vi "Write Numeric.vi"(8 "error in (no error)":errorcluster, 10 "Numeric":dbl, 11 "myChildClass in":refnum<class "myChildClass.lvclass">) -> (0 "error out":errorcluster, 3 "myChildClass out":refnum<class "myChildClass.lvclass">)   [LabVIEW 2017, in "myChildClass.lvclass"]
uses:
  myChildClass.lvclass
  myChildClass.lvclass/myChildClass.ctl
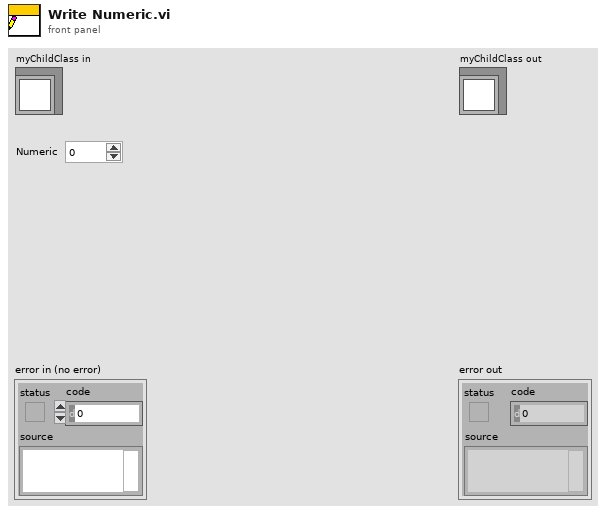
[diagram p1: front panel]
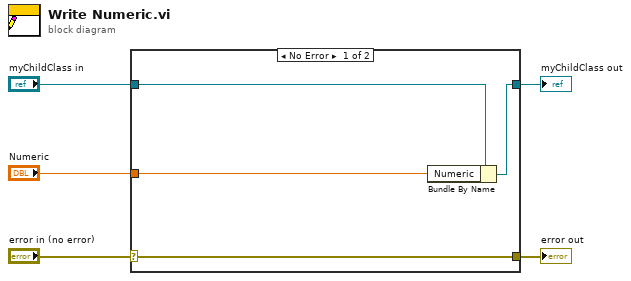
[diagram p0: block diagram]
diagram:
  n1 = case shown="No Error" "error in (no error)" {
    selector: "error in (no error)" -> [w9 w10]
    tunnel: [w9 w10] -> w4
    tunnel: [w7 w11] -> w2
    tunnel: "myChildClass in" -> [w8 w11]
    tunnel: "Numeric" -> [w6 _]
    frame No Error {
      n2 = Bundle By Name(cluster=w8, "Numeric"=w6) -> (w7:refnum<class "myChildClass.lvclass">)
    }
    frame Error {
    }
  }
  "error out" <- w4
  "myChildClass out" <- w2
